vi "Get To Add.vi"(8 "error in (no error)":errorcluster, 11 "ByRef Add in":refnum<class "ByRef Add.lvclass">) -> (0 "error out":errorcluster, 2 "To Add":dbl, 3 "ByRef Add out":refnum<class "ByRef Add.lvclass">)   [LabVIEW 2020, in "ByRef Add.lvclass"]
uses:
  ByRef Add.lvclass
  ByRef Add.lvclass/ByRef Add.ctl
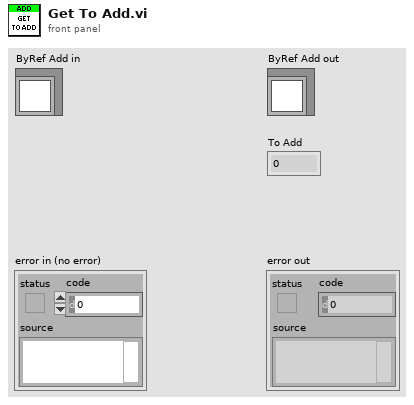
[diagram p1: front panel]
types:
  T1 = typedef "ByRef Add.lvclass/Ref Data.ctl" = cluster{"To Add":dbl}
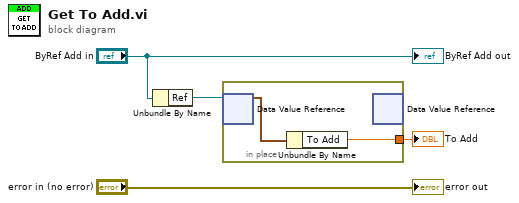
[diagram p0: block diagram]
diagram:
  n1 = Unbundle By Name("ByRef Add in") -> ("Ref"=w3:refnum<data-value>)
  n2 = in-place {
    in-place-border: [w5] -> w1
    n3 = in-place-dvr #1(w3) -> (w6:T1)  [unwired: 1 out]
    n4 = Unbundle By Name(w6) -> ("To Add"=w5:dbl)
    n5 = in-place-dvr #1() -> ()  [unwired: 1 in, 2 out]
  }
  "To Add" <- w1
  "error out" <- "error in (no error)"
  "ByRef Add out" <- "ByRef Add in"
